vi "Load Cfg.vi"(8 "error in (no error)":errorcluster, 11 "Socket in":refnum<class "Socket.lvclass">) -> (0 "error out":errorcluster, 3 "Socket out":refnum<class "Socket.lvclass">)   [LabVIEW 2018, in "Socket.lvclass"]
uses:
  Socket.lvclass
  Socket.lvclass/Socket.ctl
  State Machine/CM_State Machine.lvclass/CM_State Machine.ctl
  <vilib>/Utility/config.llb/Read Key (String).vi
  <vilib>/Utility/config.llb/Read Key (Boolean).vi
  <vilib>/Utility/config.llb/Read Key (U32).vi
  <vilib>/Utility/config.llb/NI_LVConfig.lvlib
  State Machine/CM_State Machine.lvclass
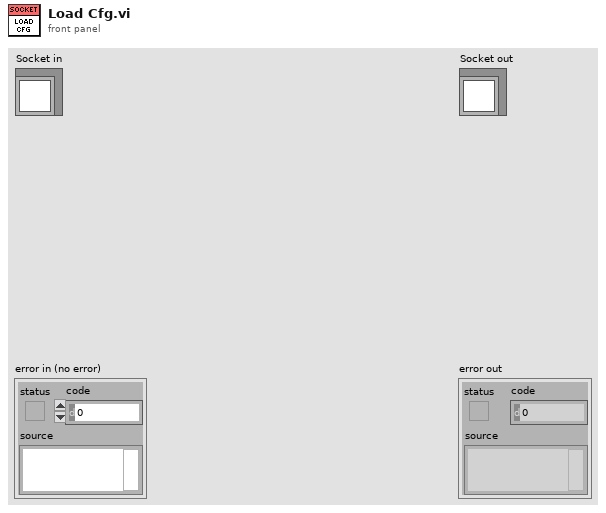
[diagram p1: front panel]
types:
  T1 = typedef "NI_LVConfig.lvlib/Config Data RefNum.ctl" = refnum<k1>
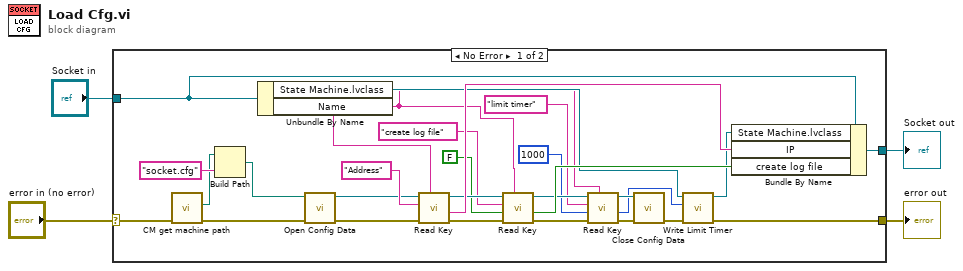
[diagram p0: block diagram]
diagram:
  n1 = case shown="No Error" "error in (no error)" {
    selector: "error in (no error)" -> [w24 w34]
    tunnel: [w13 w34] -> w3
    tunnel: [w22 w33] -> w1
    tunnel: "Socket in" -> [w25 w33]
    frame No Error {
      n2 = call "CM get machine path.vi"("error in (no error) 2"=w24) -> ("error in (no error)"=w26:errorcluster, "machine path"=w27:path)  [unwired: 9 in]
      n3 = Build Path(base path=w27, name or relative path="socket.cfg") -> (appended path=w32:path)
      n4 = Unbundle By Name(w25) -> ("State Machine.lvclass"=w16:refnum<class "CM_State Machine.lvclass">, "Name"=w7:string)
      n5 = call <vilib>:"Open Config Data.vi"("error in (no error)"=w26, "configuration file path"=w32) -> ("error out"=w28:errorcluster, "refnum"=w29:T1)  [unwired: 7 in, 1 out]
      n6 = call-poly <vilib>:"Read Key.vi"("section"=w7, "error in (no error)"=w28, "key"="Address", "refnum"=w29) -> ("error out"=w21:errorcluster, "value"=w23:string, "refnum out"=w19:T1)  [unwired: 4 in, 1 out]
      n7 = call-poly <vilib>:"Read Key.vi"("section"=w7, "error in (no error)"=w21, "default value"=FALSE, "key"="create log file", "refnum"=w19) -> ("error out"=w9:errorcluster, "value"=w20:bool, "refnum out"=w12:T1)  [unwired: 3 in, 1 out]
      n8 = call-poly <vilib>:"Read Key.vi"("section"=w7, "error in (no error)"=w9, "default value"=u32 1000, "key"="limit timer", "refnum"=w12) -> ("error out"=w10:errorcluster, "value"=w8:u32, "refnum out"=w11:T1)  [unwired: 3 in, 1 out]
      n9 = call <vilib>:"Close Config Data.vi"("error in (no error)"=w10, "refnum"=w11) -> ("error out"=w14:errorcluster)  [unwired: 8 in, 1 out]
      n10 = call "Write Limit Timer.vi"("error in (no error)"=w14, "Limit Timer"=w8, "State Machine in"=w16) -> ("error out"=w13:errorcluster, "State Machine out"=w15:refnum<class "CM_State Machine.lvclass">)  [unwired: 7 in]
      n11 = Bundle By Name(cluster=w25, "State Machine.lvclass"=w15, "IP"=w23, "create log file"=w20) -> (w22:refnum<class "Socket.lvclass">)
    }
    frame Error {
    }
  }
  "error out" <- w3
  "Socket out" <- w1
